vi "GlobalNameAngles.vi"() -> ()   [LabVIEW 2013]
panel:
  out "Global_Alt_Azh":string
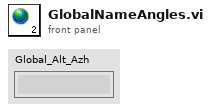
[diagram p1: front panel]
diagram:
